vi "memory_load_C_0.vi"() -> (0 "Init Data Out":fxp<+/-,32,16>[][](array[numeric]))   [LabVIEW 2020]
panel:
  # "For Initialization VI requirements and help, please read directions located on Block Diagram."
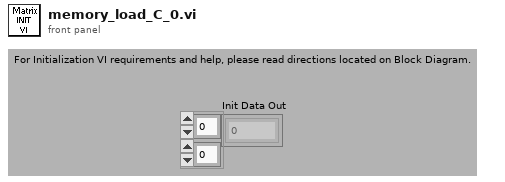
[diagram p1: front panel]
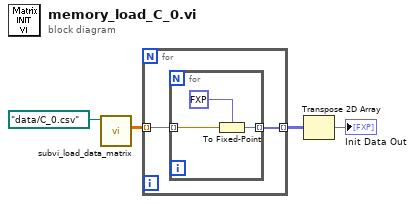
[diagram p0: block diagram]
diagram:
  n1 = call "subvi_load_data_matrix.vi"("default name"=path "data/C_0.csv") -> ("array"=w2:dbl[][])  [unwired: 10 in]
  n2 = for {
    tunnel: w2 -> [w6] mode=indexing
    tunnel: [w5] -> w1 mode=indexing
    n3 = for {
      tunnel: w6 -> [w9] mode=indexing
      tunnel: [w8] -> w5 mode=indexing
      n4 = To Fixed-Point(fixed-point type=fxp<+/-,32,16> 0.0 ("fixed-point"), number=w9) -> (fixed-point=w8:fxp<+/-,32,16>)
    }
  }
  n5 = Transpose 2D Array(2D array=w1) -> (transposed array=→"Init Data Out":fxp<+/-,32,16>[][])
